vi "ReceptionV2.vi"(5 "Nom de ressource VISA":refnum<visa-resource-name>, 6 "entrée d'erreur (pas d'erreur)":errorcluster) -> (0 "buffer de non lecture":string, 1 "Checksum OK?":bool=TRUE, 2 "Data":sgl format="%.2f", 3 "Sortie d'erreur":errorcluster caption="entrée d'erreur (pas d'erreur)", 4 "ID byte":i32)   [LabVIEW 2010]
doc: "Reception des données"
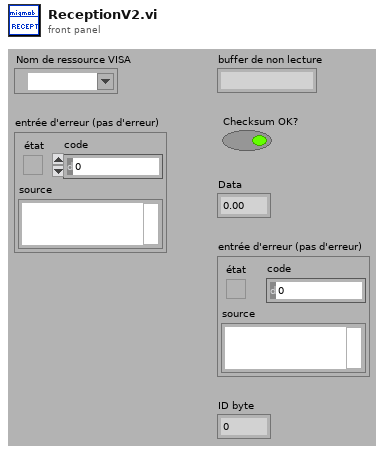
[diagram p1: front panel]
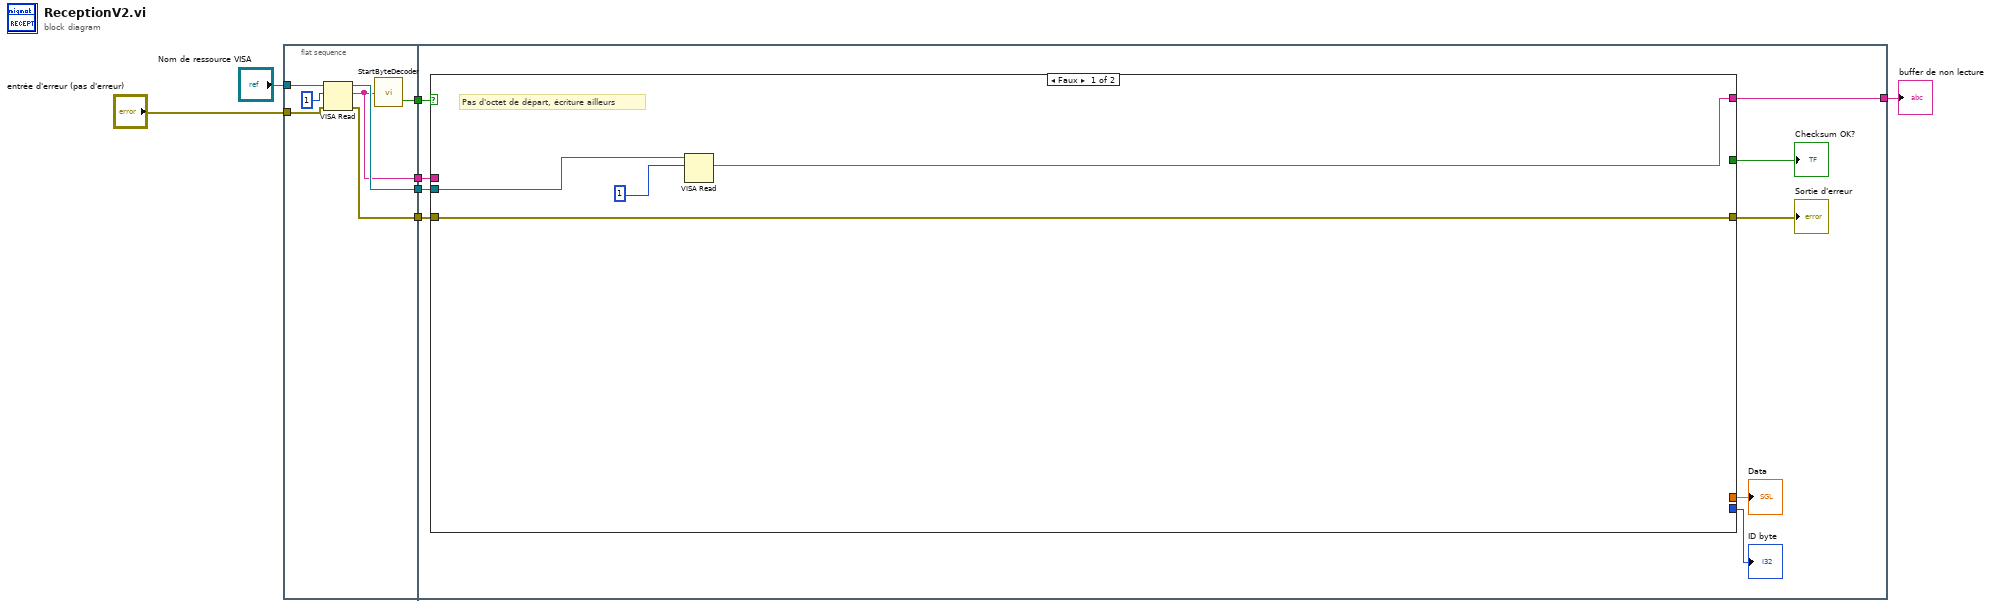
[diagram p0: block diagram]
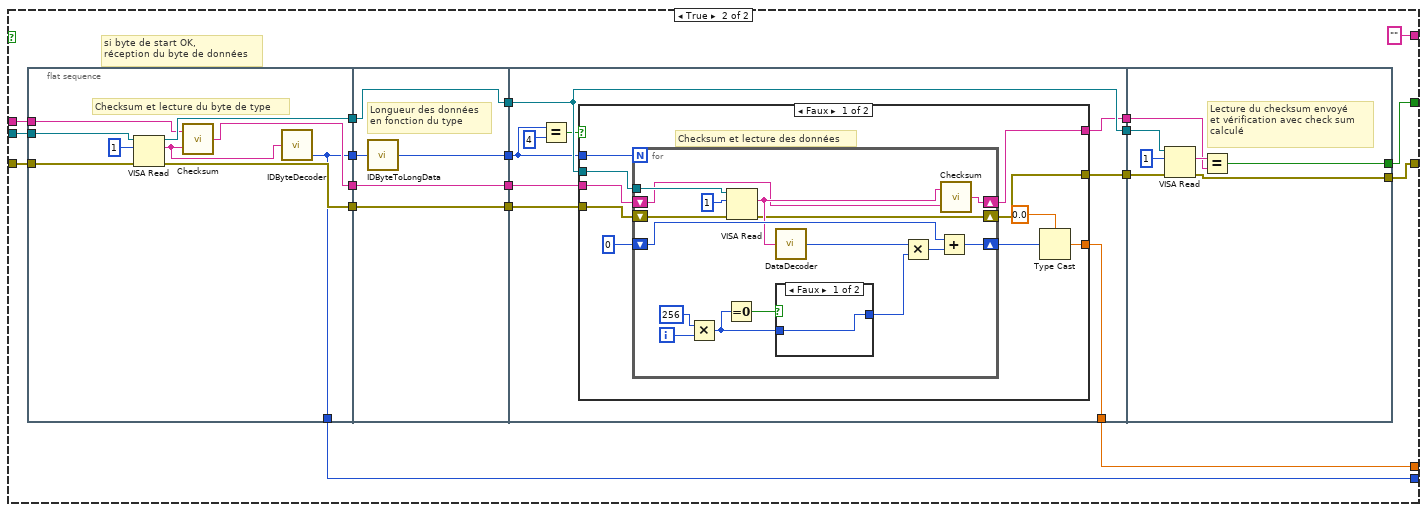
[diagram p2: hidden frame]
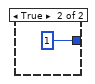
[diagram p3: hidden frame]
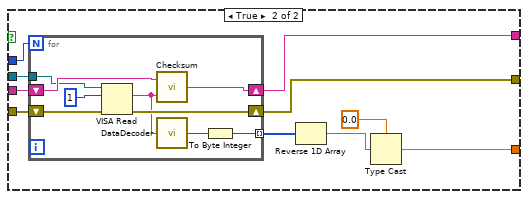
[diagram p4: hidden frame]
diagram:
  n1 = flat-sequence {
    tunnel: "Nom de ressource VISA" -> [w14]
    tunnel: "entrée d'erreur (pas d'erreur)" -> [w12]
    tunnel: [w11] -> w7
    tunnel: [w10] -> w6
    tunnel: [w9] -> w5
    tunnel: [w8] -> w4
    tunnel: w7 -> [w23]
    tunnel: w6 -> [w22]
    tunnel: w5 -> [w21]
    tunnel: w4 -> [w20]
    tunnel: [w15] -> w3
    frame #0 {
      n2 = VISA Read(VISA resource name=w14, byte count=u32 1 ("nombre d'octets"), error in (no error)=w12) -> (VISA resource name out=w10:refnum<visa-resource-name>, read buffer=w8:string, error out=w9:errorcluster)  [unwired: 1 out]
      n3 = call "StartByteDecoder.vi"("byte1"=w8) -> ("Byte Start ?"=w11:bool)  [unwired: 1 in]
    }
    frame #1 {
      n4 = case shown="Faux" w23 {
        tunnel: w22 -> [w25 w46]
        tunnel: w21 -> [w27 w45]
        tunnel: w20 -> [_ w38]
        tunnel: [_ w32] -> w19
        tunnel: [_ w31] -> w18
        tunnel: [_ w30] -> w17
        tunnel: [w27 w29] -> w16
        tunnel: [w26 "" ("read buffer")] -> w15
        frame False {
          # "Pas d'octet de départ, écriture ailleurs"
          n5 = VISA Read(VISA resource name=w25, byte count=u32 1 ("nombre d'octets")) -> (read buffer=w26:string)  [unwired: 1 in, 3 out]
        }
        frame True {
          # "si byte de start OK,\nréception du byte de données"
          n6 = flat-sequence {
            tunnel: w46 -> [w55]
            tunnel: w45 -> [w53]
            tunnel: [w47] -> w44
            tunnel: [w52] -> w42
            tunnel: [w51] -> w40
            tunnel: w38 -> [w49]
            tunnel: [w48] -> w36
            tunnel: [w47] -> w32
            tunnel: w44 -> [w60]
            tunnel: [w59] -> w43
            tunnel: w42 -> [w58]
            tunnel: [w58] -> w41
            tunnel: w40 -> [w57]
            tunnel: [w57] -> w39
            tunnel: [w56] -> w37
            tunnel: w36 -> [w56]
            tunnel: w43 -> [w63]
            tunnel: w41 -> [w67]
            tunnel: w39 -> [w69]
            tunnel: w37 -> [w68]
            tunnel: [w67] -> w35
            tunnel: [w66] -> w34
            tunnel: [w65] -> w33
            tunnel: [w64] -> w31
            tunnel: w35 -> [w122]
            tunnel: w34 -> [w121]
            tunnel: w33 -> [w119]
            tunnel: [w118] -> w30
            tunnel: [w117] -> w29
            frame #0 {
              # "Checksum et lecture du byte de type"
              n7 = VISA Read(VISA resource name=w55, byte count=u32 1 ("nombre d'octets"), error in (no error)=w53) -> (VISA resource name out=w52:refnum<visa-resource-name>, read buffer=w50:string, error out=w51:errorcluster)  [unwired: 1 out]
              n8 = call "Checksum.vi"("Byte2"=w50, "Byte1"=w49) -> ("chaîne"=w48:string)
              n9 = call "IDByteDecoder.vi"("byte1"=w50) -> ("Type de donnee (ID)"=w47:i32)  [unwired: 2 out]
            }
            frame #1 {
              # "Longueur des données\nen fonction du type"
              n10 = call "IDByteToLongData.vi"("ID Byte"=w60) -> ("Data Long"=w59:i32)
            }
            frame #2 {
              n11 = Equal?(x=w63, y=4) -> (x = y?=w61:bool)
              n12 = case shown="Faux" w61 {
                tunnel: w69 -> [w79 w103]
                tunnel: w63 -> [w78 w107]
                tunnel: w68 -> [w76 w106]
                tunnel: w67 -> [w75 w105]
                tunnel: [w74 w102] -> w66
                tunnel: [w73 w104] -> w65
                tunnel: [w70 w100] -> w64
                frame False {
                  # "Checksum et lecture des données"
                  n13 = for {
                    N: w78 -> [_]
                    tunnel: w75 -> [w95]
                    shift-right: [w87] -> w71
                    shift-left: 0 -> [w88]
                    shift-right: [w84] -> w73
                    shift-left: w76 -> [w85]
                    shift-right: [w83] -> w74
                    shift-left: w79 -> [w94]
                    i -> [w92]
                    n14 = Multiply(x=256, y=w92) -> (x*y=w80:i32)
                    n15 = Equal To 0?(x=w80) -> (x = 0?=w82:bool)
                    n16 = VISA Read(VISA resource name=w95, byte count=u32 1 ("nombre d'octets"), error in (no error)=w94) -> (read buffer=w86:string, error out=w83:errorcluster)  [unwired: 2 out]
                    n17 = call "DataDecoder.vi"("byte"=w86) -> ("Data"=w90:i32)
                    n18 = case shown="Faux" w82 {
                      tunnel: [w96 1 ("x")] -> w81
                      tunnel: w80 -> [w96 _]
                      frame False {
                      }
                      frame True {
                      }
                    }
                    n19 = Multiply(x=w90, y=w81) -> (x*y=w89:i32)
                    n20 = Add(x=w88, y=w89) -> (x+y=w87:i32)
                    n21 = call "Checksum.vi"("Byte2"=w85, "Byte1"=w86) -> ("chaîne"=w84:string)
                  }
                  n22 = Type Cast(type=sgl 0.0, x=w71) -> (*(type *) &x=w70:sgl)
                }
                frame True {
                  n23 = for {
                    N: w107 -> [_]
                    shift-right: [w116] -> w104
                    shift-left: w106 -> [w115]
                    tunnel: w105 -> [w114]
                    shift-right: [w111] -> w102
                    shift-left: w103 -> [w112]
                    tunnel: [w108] -> w99 mode=indexing
                    n24 = VISA Read(VISA resource name=w114, byte count=u32 1 ("nombre d'octets"), error in (no error)=w112) -> (read buffer=w110:string, error out=w111:errorcluster)  [unwired: 2 out]
                    n25 = call "Checksum.vi"("Byte2"=w110, "Byte1"=w115) -> ("chaîne"=w116:string)
                    n26 = call "DataDecoder.vi"("byte"=w110) -> ("Data"=w109:i32)
                    n27 = To Byte Integer(number=w109) -> (8bit integer=w108:i8)
                  }
                  n28 = Reverse 1D Array(array=w99) -> (reversed array=w98:i8[])
                  n29 = Type Cast(type=sgl 0.0, x=w98) -> (*(type *) &x=w100:sgl)
                }
              }
            }
            frame #3 {
              # "Lecture du checksum envoyé\net vérification avec check sum \ncalculé"
              n30 = VISA Read(VISA resource name=w122, byte count=u32 1 ("nombre d'octets"), error in (no error)=w121) -> (read buffer=w120:string, error out=w117:errorcluster)  [unwired: 2 out]
              n31 = Equal?(x=w120, y=w119) -> (x = y?=w118:bool)
            }
          }
        }
      }
      "ID byte" <- w19
      "Data" <- w18
      "Checksum OK?" <- w17
      "Sortie d'erreur" <- w16
    }
  }
  "buffer de non lecture" <- w3
